vi "UDSTestVI.vi"() -> ()   [LabVIEW 2021, in "Lunar UDS CAN.lvlib"]
uses:
  Lunar UDS CAN.lvlib
  Controls/UDSActions.ctl
  Controls/UDSSessionParameters.ctl
panel:
  in  "UDS Session Parameters":T1={"XNET Interface"="CAN1@nixnet", "BaudRate"=500000, "Transmit ID"=470077443, "Receive ID"=470073347} {"Receive ID" format="%x"; "Transmit ID" format="%x"}
  out "Read Data":cluster{"DataString":string, "Data":i32[]}
  in  "Tester Present":T2={"Start Tester Present"=FALSE, "Tester Present Period"=1.0}
  out "Success ?":bool
  in  "Reset Mode":u16(ring)=1 items=["Hard Reset"=1, "Key Off On Reset"=2, "Soft Reset"=3, "Enable Rapid Power Shutdown "=4, "Disable Rapid Power Shutdown"=5]
  in  "Session Type":u16(ring)=1 items=["Default Session"=1, "ECU Programming Session"=2, "ECU Extended Diagnostic Session"=3]
  in  "Data To Write":u8[](array[numeric]) format="%.0x"
  in  "ID":u16 format="%.0x"
  out "error out":errorcluster
  in  "error in (no error)":errorcluster
  in  "Action Button":bool
  in  "UDS Action":T3
  in  "Stop Button":bool
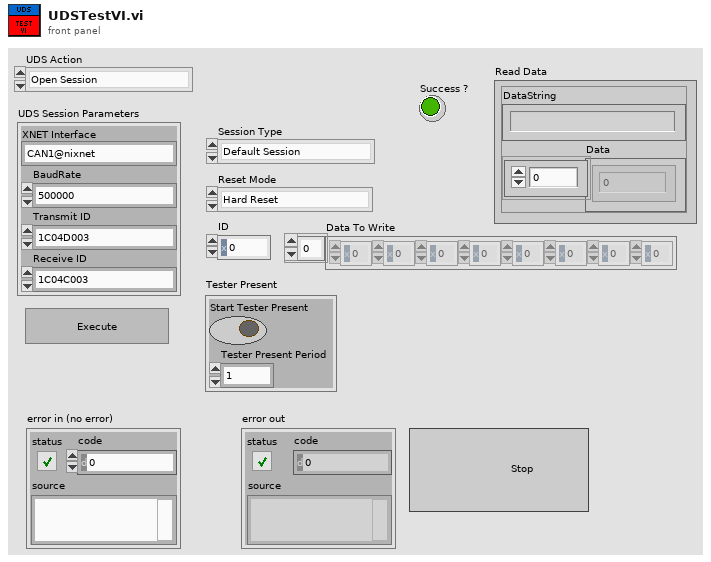
[diagram p1: front panel]
types:
  T1 = typedef "Lunar UDS CAN.lvlib/UDSSessionParameters.ctl" = cluster{"XNET Interface":string, "BaudRate":u64, "Transmit ID":i32, "Receive ID":i32}
  T2 = cluster{"Start Tester Present":bool, "Tester Present Period":dbl}
  T3 = typedef "Lunar UDS CAN.lvlib/UDSActions.ctl" = enum16{"Open Session", "Connect To Diagnostic Session", "Send Tester Present", "ECU Reset", "Write String Data", "Write Byte Data", "Read Data", "Close Session", "Close All Sessions"}
  T4 = typedef "Lunar UDS CAN.lvlib/UDSReadData.ctl" = cluster{"DataString":string, "Data":i32[]}
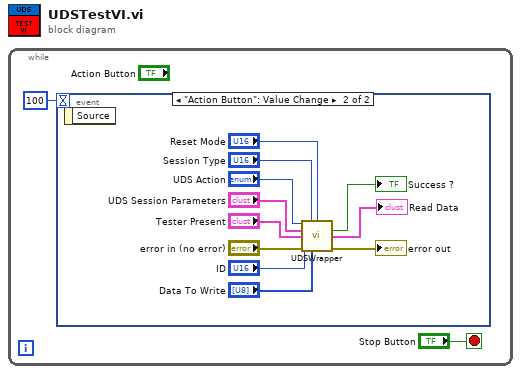
[diagram p0: block diagram]
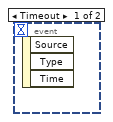
[diagram p2: hidden frame]
diagram:
  n1 = while {
    stop <- "Stop Button" stop-if-true
    n2 = event shown="[1] \"Action Button\": Value Change" {
      selector: _ -> [_ _]
      dyn-events: _ -> [_ _]
      timeout: 100 -> [_ _]
      event Timeout {
        n3 = event-data() -> ()  [unwired: 1 in, 3 out]
      }
      event "Action Button": Value Change {
        n4 = event-data() -> ()  [unwired: 1 in, 1 out]
        n5 = call "UDSWrapper.vi"("UDS Action"="UDS Action", "Session Type"="Session Type", "Reset Mode"="Reset Mode", "UDS Session Parameters"="UDS Session Parameters", "Tester Present"="Tester Present", "ID"="ID", "error in (no error)"="error in (no error)", "Byte Data To Write"="Data To Write") -> ("Success ?"=→"Success ?":bool, "Read Data"=→"Read Data":T4, "error out"=→"error out":errorcluster)  [unwired: 5 in]
      }
    }
  }
